vi "SetTimeStampToTimeCtrl.vi"(10 "time":timestamp, 11 "ref in":refnum<vi>) -> (3 "ref out":refnum<vi>)   [LabVIEW 2018, in "Library-Ctrl.lvlib"]
uses:
  Library-Ctrl.lvlib
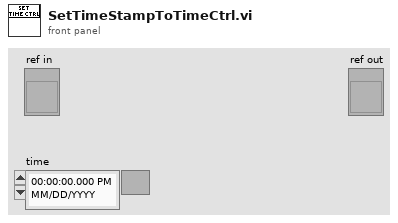
[diagram p1: front panel]
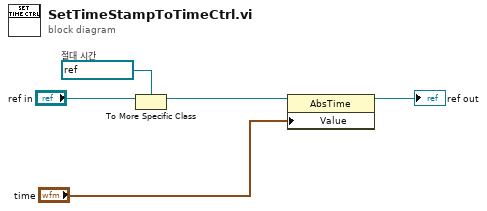
[diagram p0: block diagram]
diagram:
  w4 = refnum<vi> refnum  # 절대 시간
  n1 = To More Specific Class(target class=w4, reference="ref in") -> (specific class reference=w3:refnum<vi>)  [unwired: 1 in, 1 out]
  n2 = property class="AbsTime"(reference=w3, "Value"="time") -> (reference out=→"ref out":refnum<vi>)  [unwired: 1 in, 1 out]
